vi "Prime95BCameraSimpleOperationACQ.vi"(8 "error in (no error)":errorcluster, 11 "Config In":T1 {"Hardware Configuration"."Lasers Configuration"."SettingValues"."785 Power" format="%.1f"; "Hardware Configuration"."Lasers Configuration"."SettingValues"."647 Power" format="%.1f"; "Hardware Configuration"."Lasers Configuration"."SettingValues"."561 Power" format="%.1f"}) -> (0 "error out":errorcluster, 3 "Config Out":T1 {"Hardware Configuration"."Lasers Configuration"."SettingValues"."785 Power" format="%.1f"; "Hardware Configuration"."Lasers Configuration"."SettingValues"."647 Power" format="%.1f"; "Hardware Configuration"."Lasers Configuration"."SettingValues"."561 Power" format="%.1f"})   [LabVIEW 2019]
uses:
  Settings/System Running Settings.ctl
  HardwareAdapter/Support/Hardware Configuration.ctl
  HardwareAdapter/Support/Camera Configuration.ctl
  E:/DevHardSoftware/MMicroscopy/HardwareAdapter/Camera/Dependencies/PVCamNET.dll
  HardwareAdapter/Camera/Dependencies/PVCamNET.dll
  <vilib>/vision/Image Controls.llb/IMAQ Image.ctl
  E:/DevHardSoftware/MMicroscopy/HardwareAdapter/Lasers/Dependencies/Oxxius_Boxx.dll
  HardwareAdapter/Lasers/Dependencies/Oxxius_Boxx.dll
  Logging/Logging Configuration.ctl
  controls/DeviceStatusCtl.ctl
  controls/CallBack Refs.ctl
  Logging/Logging.lvlib
  Settings/Settings.lvlib
panel:
  out "8 Bit Histogram":i32[](graph)
  in  "start":bool
  in  "stop":bool
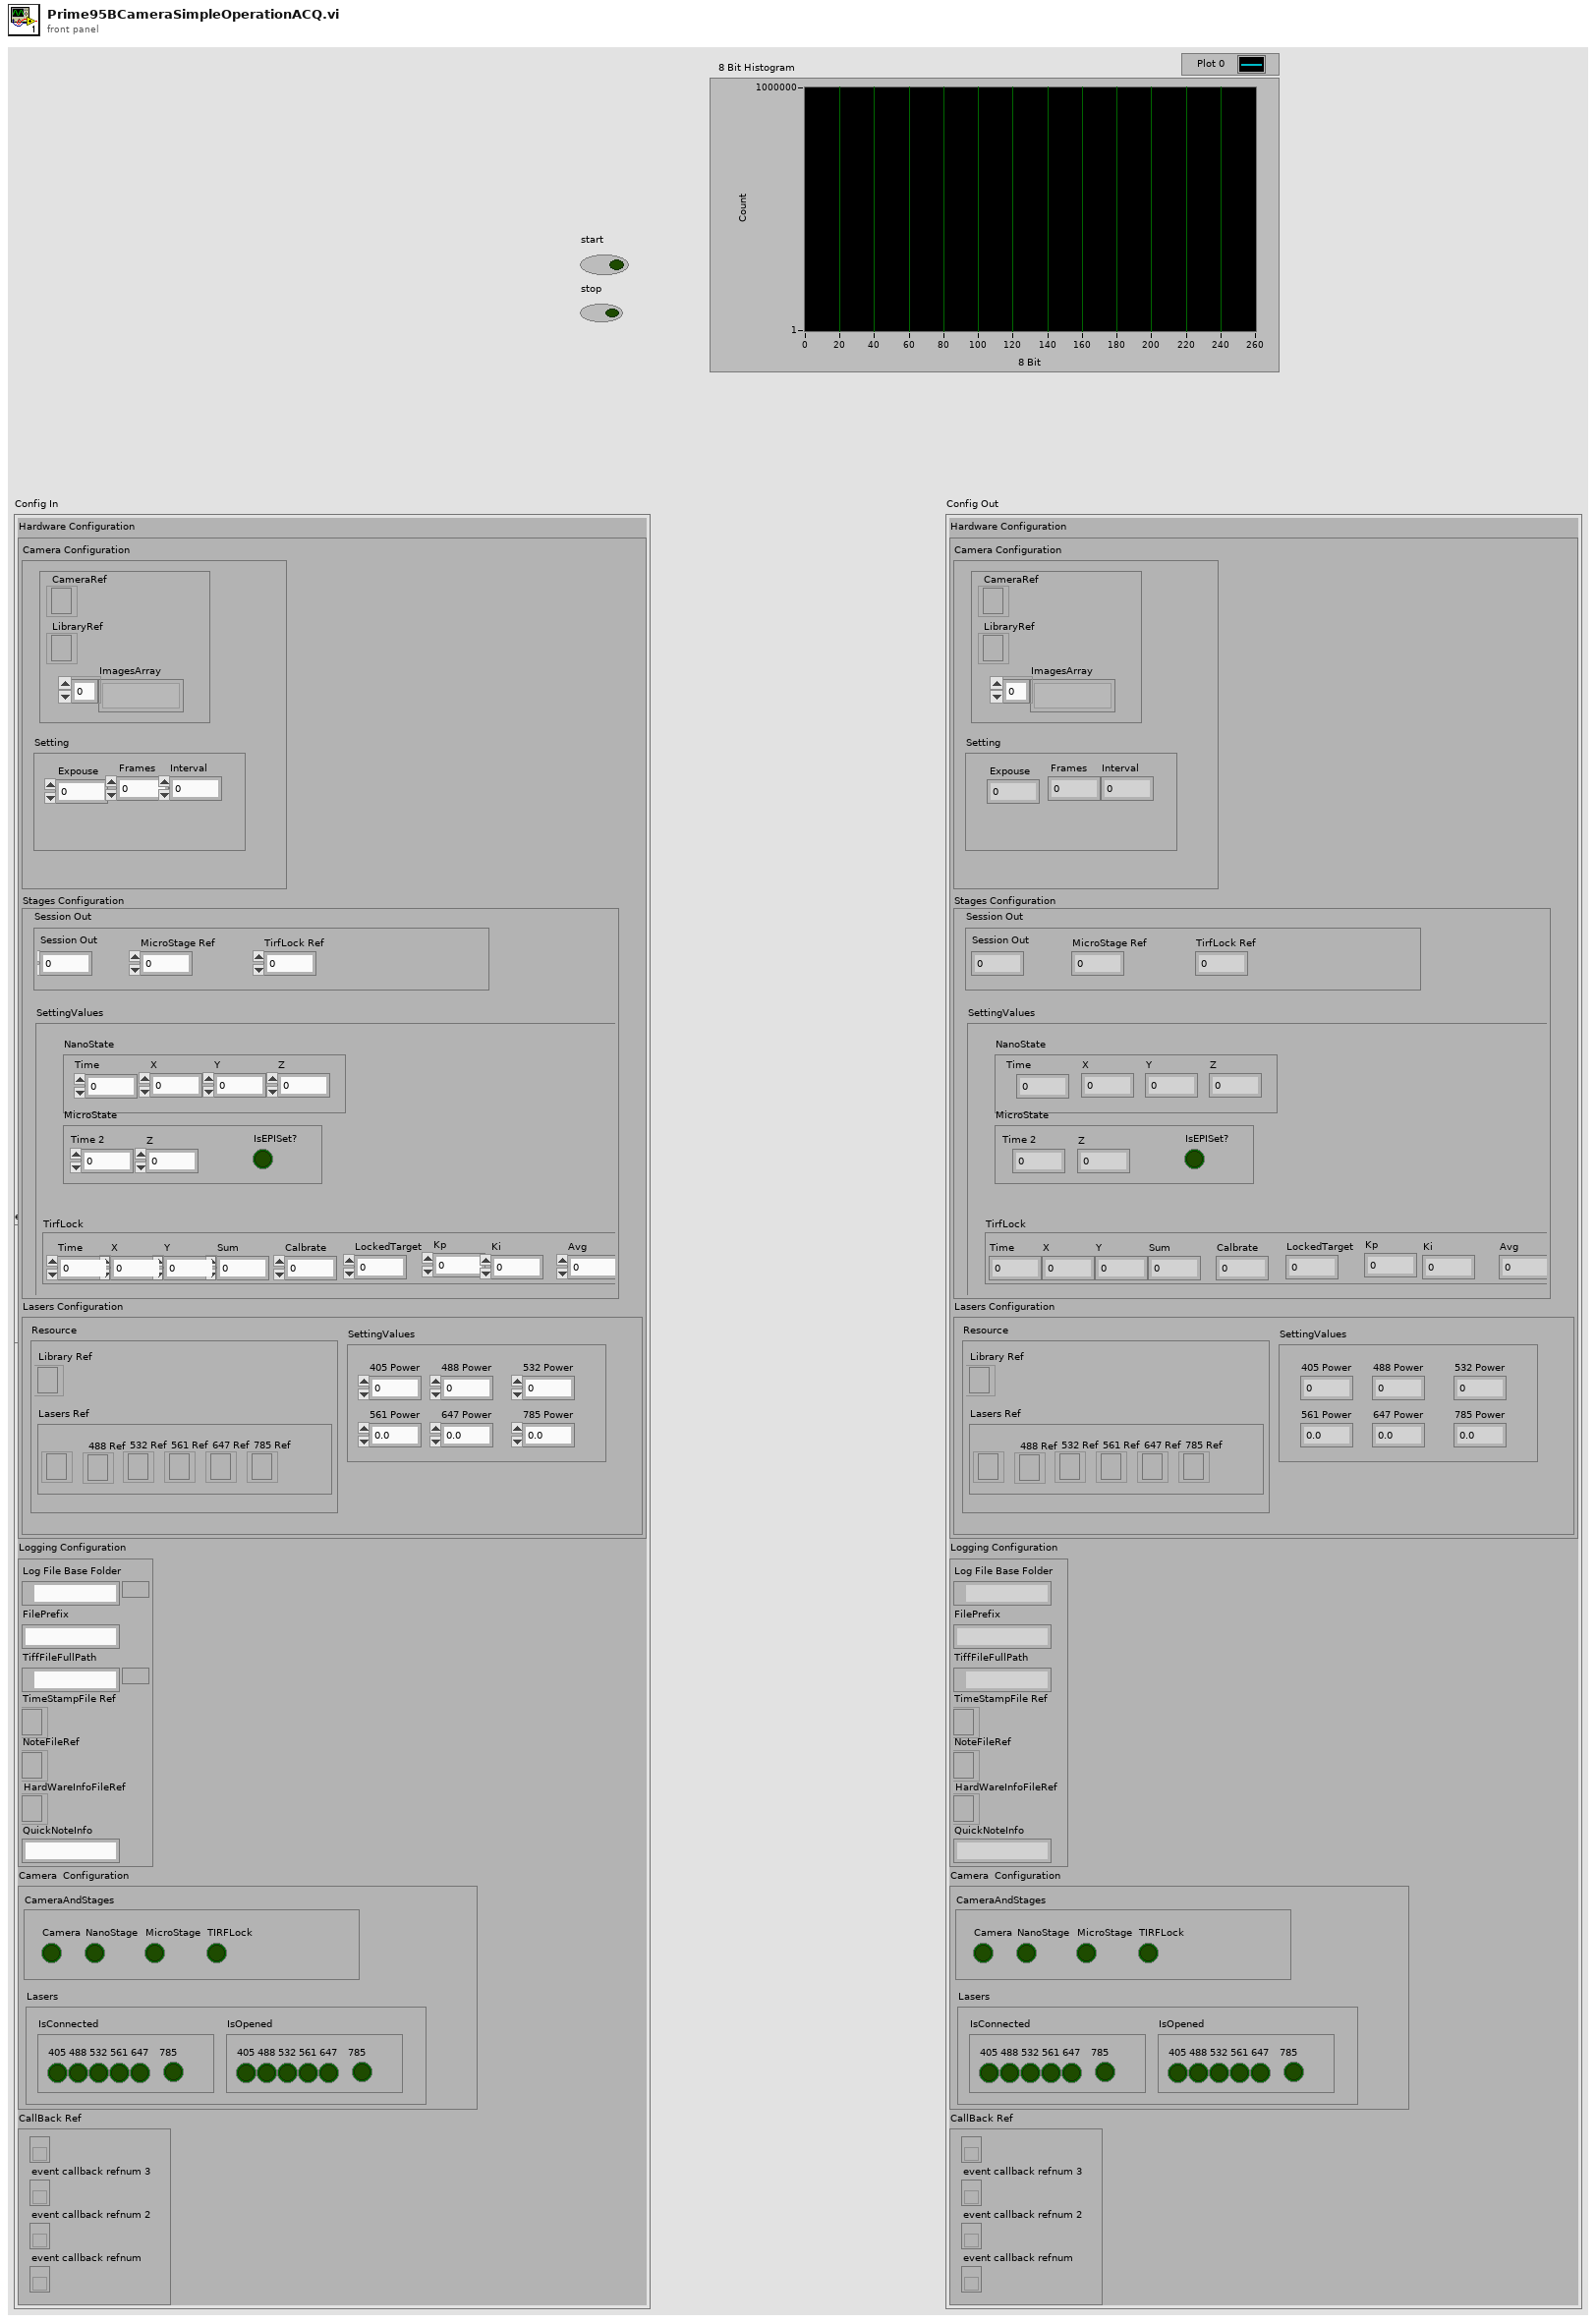
[diagram p1: front panel]
types:
  T1 = typedef "Settings.lvlib/System Running Settings.ctl" = cluster{"Hardware Configuration":T2, "Logging Configuration":T5, "HardWare Status":cluster{"CameraAndStages":T6, "Lasers":cluster{"IsConnected":cluster{"405":bool, "488":bool, "532":bool, "561":bool, "647":bool, "785":bool}, "IsOpened":cluster{"405":bool, "488":bool, "532":bool, "561":bool, "647":bool, "785":bool}}}, "CallBack Ref":T7}
  T2 = typedef "Hardware Configuration.ctl" = cluster{"Camera Configuration":T3, "Stages Configuration":cluster{"Resource":cluster{"NanoStage Ref":i32, "MicroStage Ref":i32, "TirfLock Ref":i32}, "SettingValues":cluster{"NanoState":cluster{"Time":dbl, "X":dbl, "Y":dbl, "Z":dbl}, "MicroState":cluster{"Time 2":dbl, "Z":dbl, "IsEPISet?":bool}, "TirfLock":cluster{"Time":dbl, "X":dbl, "Y":dbl, "Sum":dbl, "Calbrate":dbl, "LockedTarget":dbl, "Kp":dbl, "Ki":dbl, "Avg":dbl}}}, "Lasers Configuration":cluster{"SettingValues":cluster{"405 Power":sgl, "488 Power":sgl, "532 Power":sgl, "561 Power":sgl, "647 Power":sgl, "785 Power":sgl}, "Resource":cluster{"Library Ref":refnum<k24>, "Lasers Ref":cluster{"405 Ref":refnum<k24>, "488 Ref":refnum<k24>, "532 Ref":refnum<k24>, "561 Ref":refnum<k24>, "647 Ref":refnum<k24>, "785 Ref":refnum<k24>}}}}
  T3 = typedef "Camera Configuration.ctl" = cluster{"Setting":cluster{"Expouse":dbl, "Frames":dbl, "Interval":dbl}, "Resource":cluster{"CameraRef":refnum<k24>, "LibraryRef":refnum<k24>, "ImagesArray":T4[]}}
  T4 = typedef "IMAQ Image.ctl" = refnum<image>
  T5 = typedef "Logging.lvlib/Logging Configuration.ctl" = cluster{"Log File Base Folder":path, "FilePrefix":string, "TiffFileFullPath":path, "TimeStampFile Ref":refnum<file>, "NoteFileRef":refnum<file>, "HardWareInfoFileRef":refnum<file>, "QuickNoteInfo":string}
  T6 = typedef "DeviceStatusCtl.ctl" = cluster{"Camera":bool, "NanoStage":bool, "MicroStage":bool, "TIRFLock":bool}
  T7 = typedef "CallBack Refs.ctl" = cluster{"event callback refnum":refnum<k27>, "event callback refnum 2":refnum<k27>, "event callback refnum 3":refnum<k27>, "event callback refnum 4":refnum<k27>}
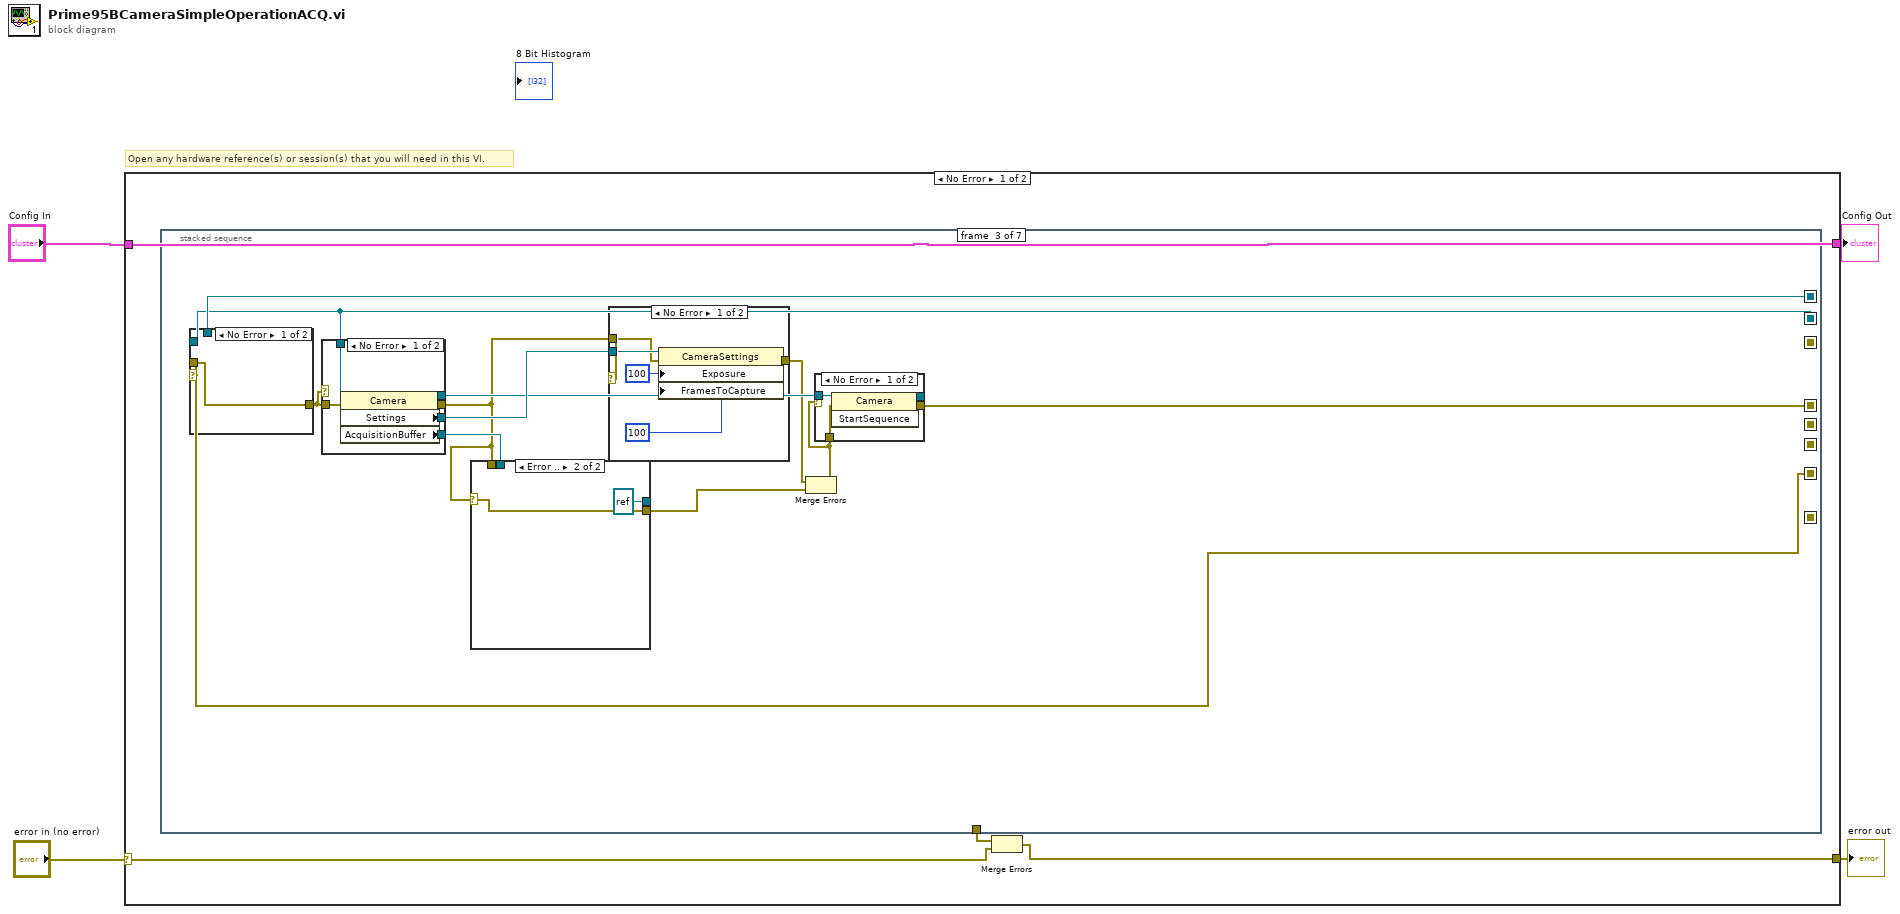
[diagram p0: block diagram]
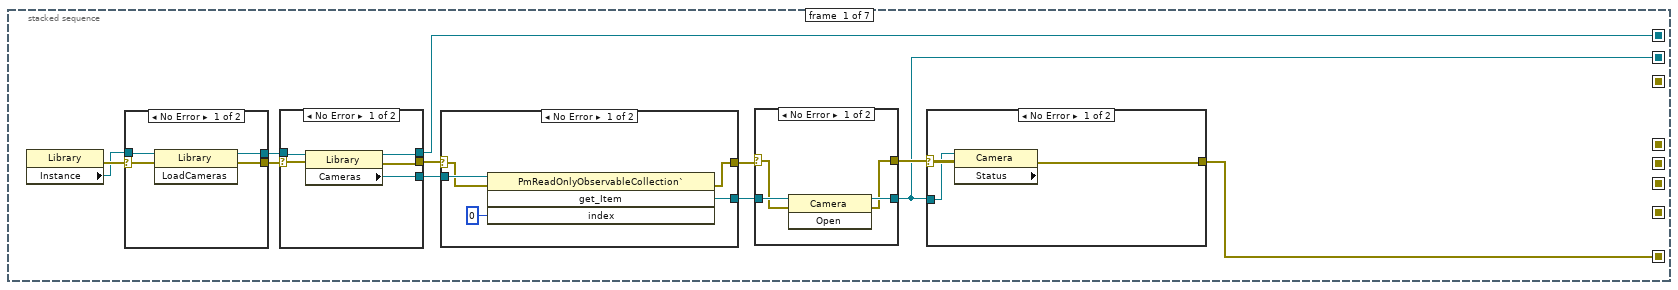
[diagram p2: hidden frame]
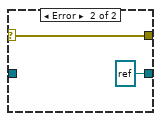
[diagram p4: hidden frame]
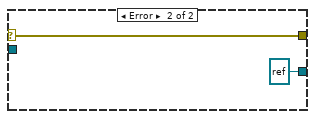
[diagram p5: hidden frame]
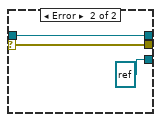
[diagram p6: hidden frame]
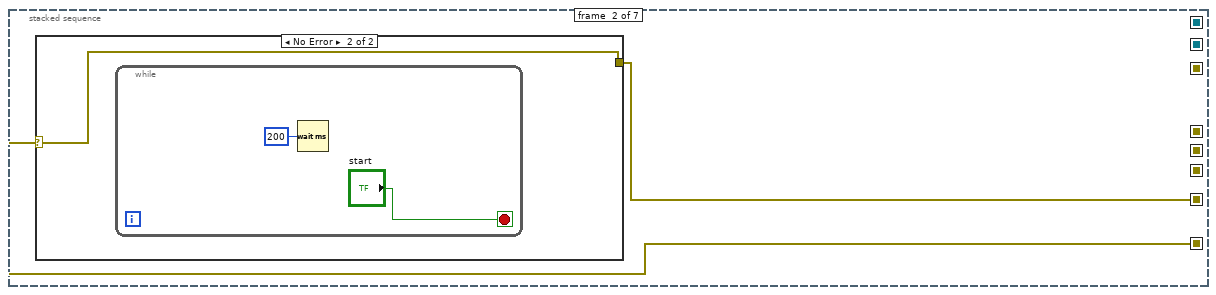
[diagram p8: hidden frame]
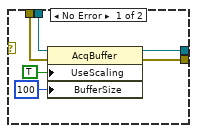
[diagram p12: hidden frame]
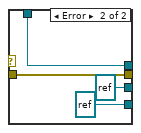
[diagram p13: hidden frame]
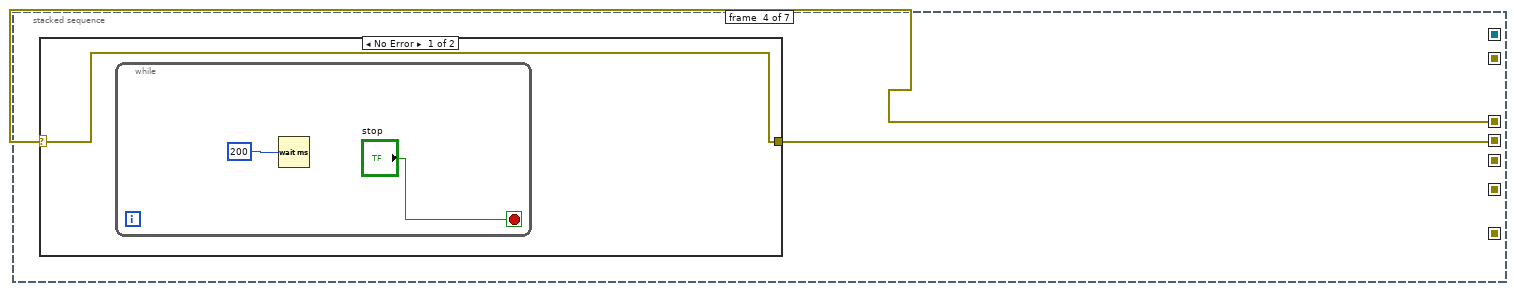
[diagram p15: hidden frame]
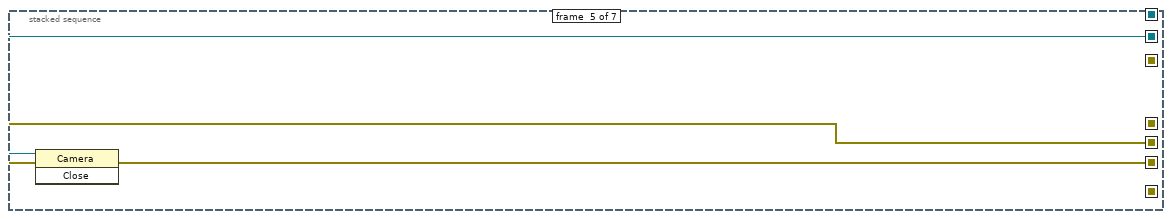
[diagram p17: hidden frame]
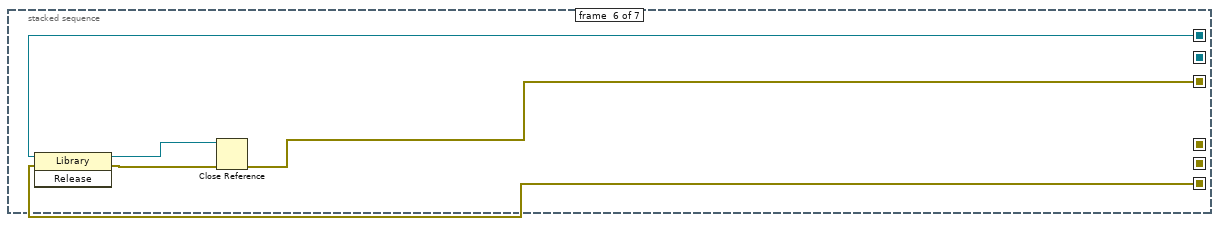
[diagram p18: hidden frame]
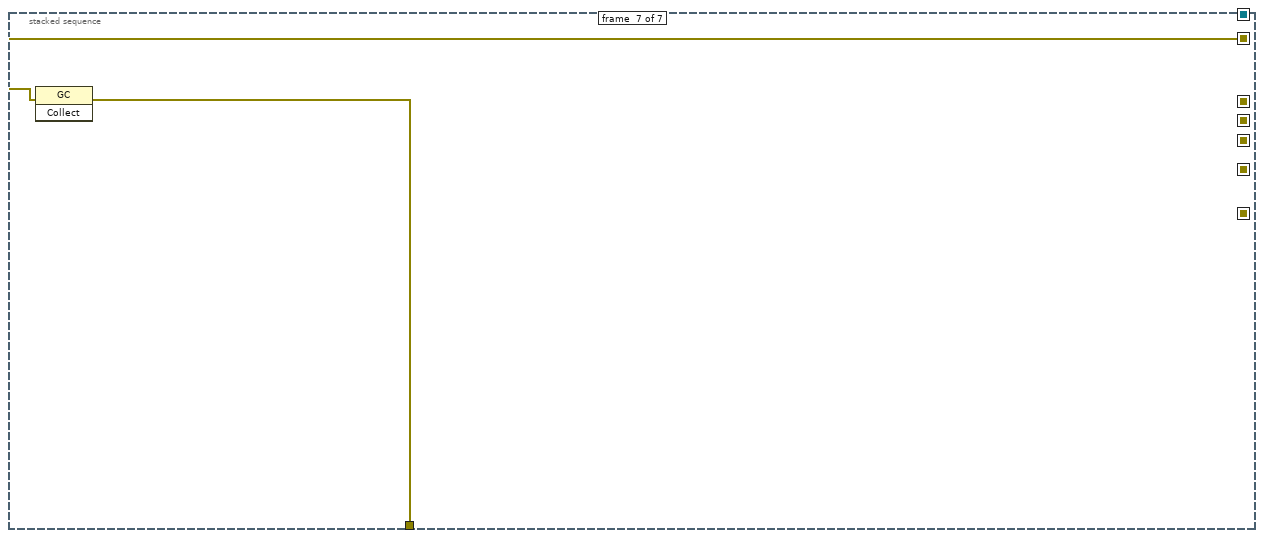
[diagram p19: hidden frame]
diagram:
  # "Open any hardware reference(s) or session(s) that you will need in this VI."
  n1 = case shown="No Error" "error in (no error)" {
    selector: "error in (no error)" -> [w6 w118]
    tunnel: [w5 w118] -> w3
    tunnel: "Config In" -> [w8 w119]
    tunnel: [w8 w119] -> w1
    frame No Error {
      n2 = stacked-sequence {
        seq-local: [w10 _ _ _ _ _ _] -> [_ w53 _ _ _ _ _]
        seq-local: [w9 _ _ _ _ _ _] -> [_ _ w66 _ w110 _ _]
        seq-local: [w12 _ _ _ _ _ _] -> [_ _ w69 _ _ w114 _]
        seq-local: [_ _ w58 _ _ _ _] -> [_ _ _ w103 _ _ _]
        seq-local: [_ _ _ _ w109 _ _] -> [_ _ _ _ _ w113 _]
        seq-local: [_ _ _ _ _ w111 _] -> [_ _ _ _ _ _ w117]
        seq-local: [_ w52 _ _ _ _ _] -> [_ _ w62 _ _ _ _]
        seq-local: [_ _ _ w102 _ _ _] -> [_ _ _ _ w108 _ _]
        tunnel: [_ _ _ _ _ _ w116] -> w7
        frame #0 {
          n3 = property class="Library"() -> (error out=w20:errorcluster, "Instance"=w17:refnum<k24>)  [unwired: 2 in, 1 out]
          n4 = case shown="No Error" w20 {
            selector: w20 -> [w47 w51]
            tunnel: [w48 w51] -> w18
            tunnel: [w49 w50] -> w19
            tunnel: w17 -> [w46 w50]
            frame No Error {
              n5 = invoke class="Library" method="LoadCameras"(reference=w46, error in=w47) -> (reference out=w49:refnum<k24>, error out=w48:errorcluster)  [unwired: 1 in, 1 out]
            }
            frame Error {
            }
          }
          n6 = case shown="No Error" w18 {
            selector: w18 -> [w42 w45]
            tunnel: [w39 w45] -> w14
            tunnel: w19 -> [w41 w44]
            tunnel: [w40 w44] -> w12
            tunnel: [w38 refnum<k24> refnum ("Cameras")] -> w16
            frame No Error {
              n7 = property class="Library"(reference=w41, error in=w42) -> (reference out=w40:refnum<k24>, error out=w39:errorcluster, "Cameras"=w38:refnum<k24>)
            }
            frame Error {
            }
          }
          n8 = case shown="No Error" w14 {
            selector: w14 -> [w32 w37]
            tunnel: w16 -> [w35 _]
            tunnel: [w33 refnum<k24> refnum ("get_Item")] -> w15
            tunnel: [w31 w37] -> w13
            frame No Error {
              n9 = invoke class="PmReadOnlyObservableCollection`" method="get_Item"(reference=w35, error in=w32, "index"=0) -> (error out=w31:errorcluster, "get_Item"=w33:refnum<k24>)  [unwired: 1 in, 2 out]
            }
            frame Error {
            }
          }
          n10 = case shown="No Error" w13 {
            selector: w13 -> [w26 w30]
            tunnel: [w25 w30] -> w11
            tunnel: w15 -> [w28 _]
            tunnel: [w27 refnum<k24> refnum ("get_Item")] -> w9
            frame No Error {
              n11 = invoke class="Camera" method="Open"(reference=w28, error in=w26) -> (reference out=w27:refnum<k24>, error out=w25:errorcluster)  [unwired: 1 in, 1 out]
            }
            frame Error {
            }
          }
          n12 = case shown="No Error" w11 {
            selector: w11 -> [w22 w24]
            tunnel: [w21 w24] -> w10
            tunnel: w9 -> [w23 _]
            frame No Error {
              n13 = property class="Camera" props=["Status"](reference=w23, error in=w22) -> (error out=w21:errorcluster)  [unwired: 2 out]
            }
            frame Error {
            }
          }
        }
        frame #1 {
          n14 = case shown="No Error" w53 {
            selector: w53 -> [w54 w55]
            tunnel: [w54 w55] -> w52
            frame Error {
            }
            frame No Error {
              n15 = while {
                stop <- "start" stop-if-true
                n16 = Wait (ms)(milliseconds to wait=u32 200) -> ()  [unwired: 1 out]
              }
            }
          }
        }
        frame #2 {
          n17 = case shown="No Error" w62 {
            tunnel: w69 -> [_ _]
            tunnel: [w100 w101] -> w61
            tunnel: w66 -> [_ _]
            tunnel: w62 -> [w100 w101]
            frame No Error {
            }
            frame Error {
            }
          }
          n18 = case shown="No Error" w61 {
            tunnel: [w95 refnum<k24> refnum ("Settings")] -> w68
            tunnel: [w94 refnum<k24> refnum ("AcquisitionBuffer")] -> w67
            tunnel: w61 -> [w93 w99]
            tunnel: w66 -> [w92 w98]
            tunnel: [w91 w98] -> w65
            tunnel: [w90 w99] -> w60
            frame No Error {
              n19 = property class="Camera"(reference=w92, error in=w93) -> (reference out=w91:refnum<k24>, error out=w90:errorcluster, "Settings"=w95:refnum<k24>, "AcquisitionBuffer"=w94:refnum<k24>)
            }
            frame Error {
            }
          }
          n20 = case shown="Error .." w60 {
            selector: w60 -> [_ w89]
            tunnel: w67 -> [w87 _]
            tunnel: w60 -> [w85 _]
            tunnel: [w84 w89] -> w63
            tunnel: [w82 refnum<k24> refnum ("AcquisitionBuffer")] -> _
            frame No Error {
              n21 = property class="AcqBuffer"(reference=w87, error in=w85, "UseScaling"=TRUE, "BufferSize"=100) -> (reference out=w82:refnum<k24>, error out=w84:errorcluster)
            }
            frame Error {
            }
          }
          n22 = case shown="No Error" w60 {
            tunnel: w68 -> [w80 _]
            tunnel: [w79 w81] -> w64
            tunnel: w60 -> [w78 w81]
            frame No Error {
              n23 = property class="CameraSettings"(reference=w80, error in=w78, "Exposure"=u32 100, "FramesToCapture"=u16 100) -> (error out=w79:errorcluster)  [unwired: 1 out]
            }
            frame Error {
            }
          }
          n24 = Merge Errors(w64, w63) -> (w59:errorcluster)
          n25 = case shown="No Error" w59 {
            selector: w59 -> [_ w75]
            tunnel: w65 -> [w73 w74]
            tunnel: [w72 w75] -> w58
            tunnel: [w71 w74] -> _
            tunnel: w59 -> [w70 _]
            frame No Error {
              n26 = invoke class="Camera" method="StartSequence"(reference=w73, error in=w70) -> (reference out=w71:refnum<k24>, error out=w72:errorcluster)  [unwired: 1 in, 1 out]
            }
            frame Error {
            }
          }
        }
        frame #3 {
          n27 = case shown="No Error" w103 {
            selector: w103 -> [w104 w107]
            tunnel: [w104 w107] -> w102
            frame No Error {
              n28 = while {
                stop <- "stop" stop-if-true
                n29 = Wait (ms)(milliseconds to wait=u32 200) -> ()  [unwired: 1 out]
              }
            }
            frame Error {
            }
          }
        }
        frame #4 {
          n30 = invoke class="Camera" method="Close"(reference=w110, error in=w108) -> (error out=w109:errorcluster)  [unwired: 1 in, 2 out]
        }
        frame #5 {
          n31 = invoke class="Library" method="Release"(reference=w114, error in=w113) -> (reference out=w115:refnum<k24>, error out=w112:errorcluster)  [unwired: 1 in, 1 out]
          n32 = Close Reference(reference=w115, error in (no error)=w112) -> (error out=w111:errorcluster)
        }
        frame #6 {
          n33 = invoke class="GC" method="Collect"(error in=w117) -> (error out=w116:errorcluster)  [unwired: 2 in, 2 out]
        }
      }
      n34 = Merge Errors(w7, w6) -> (w5:errorcluster)
    }
    frame Error {
    }
  }
  "error out" <- w3
  "Config Out" <- w1
